vi "Swap CS with DDS.vi"(6 "Variant in":variant, 7 "Shift Pressed?":bool, 8 "error in (no error)":errorcluster, 10 "QD Combo Box Ref":refnum<vi>, 11 "QD Launch VI Ref":refnum<vi>) -> (0 "error out":errorcluster, 4 "Variant out":variant)   [LabVIEW 2017]
doc: "PLUGIN_DESCRIPTION: Replaces selected Case Structure with Diagram Disable Structure. Based on SAPHIR_DisableCode.vi from https://forums.ni.com/t5/SAPHIR-Toolkits-Documents/ViBox-Quick-Drop-datasheet/ta-p/3507939?profile.language=en\nPLUGIN_DEFAULT_SHORTCUT:"
uses:
  <userlib>/_LAVACR/Scripting Tools/Scripting Tools.lvlib
panel:
  in  "Undo Name":string="DisableCode"
  # "Created by https://github.com/Zieleslaw/, based on:"
  # "More informations on : https://decibel.ni.com/content/groups/saphir-toolkit"
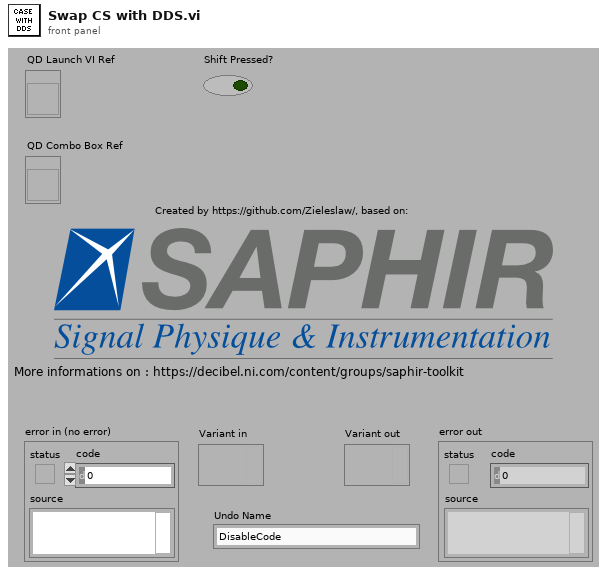
[diagram p1: front panel]
types:
  T1 = enum16{"Case Structure", "Stacked Sequence", "Event Structure", "Diagram Disable", "Conditional Disable", "While Loop", "For Loop", "Inplace Structure"}
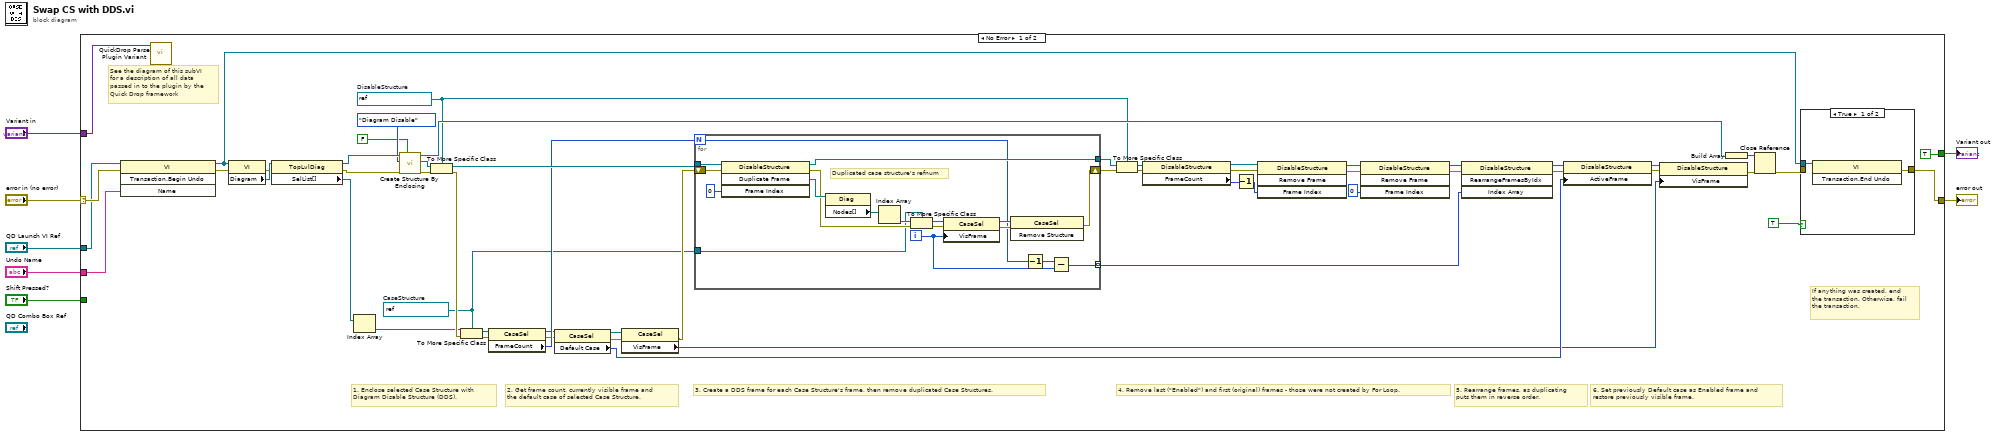
[diagram p0: block diagram]
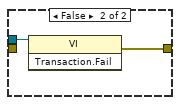
[diagram p2: hidden frame]
diagram:
  n1 = case shown="No Error" "error in (no error)" {
    selector: "error in (no error)" -> [w53 w85]
    tunnel: [w50 w85] -> w6
    tunnel: "QD Launch VI Ref" -> [w52 _]
    tunnel: "Variant in" -> [w54 _]
    tunnel: "Undo Name" -> [w51 _]
    tunnel: [TRUE _] -> w2
    tunnel: "Shift Pressed?" -> [_ _]
    frame No Error {
      w8 = refnum<vi> refnum  # CaseStructure
      w9 = refnum<vi> refnum  # DisableStructure
      # "6. Set previously Default case as Enabled frame and \nrestore previously visible frame."
      # "5. Rearrange frames, as duplicating \nputs them in reverse order."
      # "4. Remove last (\"Enabled\") and first (original) frames - those were not created by For Loop."
      # "3. Create a DDS frame for each Case Structure's frame, then remove duplicated Case Structures."
      # "2. Get frame count, currently visible frame and\nthe default case of selected Case Structure."
      # "1. Enclose selected Case Structure with\nDiagram Disable Structure (DDS)."
      # "If anything was created, end the transaction. Otherwise, fail the transaction."
      # "See the diagram of this subVI for a description of all data passed in to the plugin by the Quick Drop framework"
      n2 = invoke class="VI" method="Transaction.Begin Undo"(reference=w52, error in=w53, "Name"=w51) -> (reference out=w58:refnum<vi>, error out=w61:errorcluster)  [unwired: 1 in, 2 out]
      n3 = call <vilib>:"QuickDrop Parse Plugin Variant.vi"("QDKS Variant in"=w54) -> ()  [unwired: 12 in, 3 out]
      n4 = property class="VI"(reference=w58, error in=w61) -> (error out=w55:errorcluster, "Diagram"=w56:refnum<vi>)  [unwired: 1 out]
      n5 = property class="TopLvlDiag"(reference=w56, error in=w55) -> (reference out=w57:refnum<vi>, error out=w60:errorcluster, "SelList[]"=w48:refnum<vi>[])
      n6 = Index Array(array=w48) -> (element=w10:refnum<vi>)  [unwired: 1 in]
      n7 = call <userlib>:"Create Structure By Enclosing.vi"("Select everything except terminals ?"=FALSE, "error in (no error)"=w60, "Structure Type"=T1."Diagram Disable", "Diagram In"=w57) -> ("error out"=w44:errorcluster, "Structure Out"=w45:refnum<vi>, "Diagram Out"=w11:refnum<vi>)  [unwired: 5 in]
      n8 = To More Specific Class(target class=w9, reference=w45, error in=w44) -> (specific class reference=w42:refnum<vi>, error out=w32:errorcluster)
      n9 = To More Specific Class(target class=w8, reference=w10, error in=w32) -> (specific class reference=w40:refnum<vi>, error out=w33:errorcluster)
      n10 = property class="CaseSel"(reference=w40, error in=w33) -> (reference out=w38:refnum<vi>, error out=w37:errorcluster, "FrameCount"=w39:i32)
      n11 = property class="CaseSel"(reference=w38, error in=w37) -> (reference out=w35:refnum<vi>, error out=w34:errorcluster, "Default Case"=w36:i32)
      n12 = property class="CaseSel"(reference=w35, error in=w34) -> (error out=w12:errorcluster, "VisFrame"=w18:u32)  [unwired: 1 out]
      n13 = for {
        N: w39 -> [w67]
        tunnel: [w70] -> w30
        tunnel: w42 -> [w80]
        shift-right: [w71] -> w29
        shift-left: w12 -> [w79]
        tunnel: [w64] -> w17 mode=indexing
        tunnel: w8 -> [w63]
        i -> [w66]
        # "Duplicated case structure's refnum"
        n14 = invoke class="DisableStructure" method="Duplicate Frame"(reference=w80, error in=w79, "Frame Index"=u32 0) -> (reference out=w70:refnum<vi>, error out=w69:errorcluster, "Duplicate Frame"=w78:refnum<vi>)  [unwired: 1 in, 1 out]
        n15 = property class="Diag"(reference=w78) -> ("Nodes[]"=w77:refnum<vi>[])  [unwired: 1 in, 2 out]
        n16 = Index Array(array=w77) -> (element=w76:refnum<vi>)  [unwired: 1 in]
        n17 = To More Specific Class(target class=w63, reference=w76, error in=w69) -> (specific class reference=w75:refnum<vi>, error out=w74:errorcluster)
        n18 = property class="CaseSel"(reference=w75, error in=w74, "VisFrame"=w66) -> (reference out=w73:refnum<vi>, error out=w72:errorcluster)
        n19 = invoke class="CaseSel" method="Remove Structure"(reference=w73, error in=w72) -> (error out=w71:errorcluster)  [unwired: 1 in, 2 out]
        n20 = Decrement(x=w67) -> (x-1=w65:i32)
        n21 = Subtract(x=w65, y=w66) -> (x-y=w64:i32)
      }
      n22 = To More Specific Class(target class=w9, reference=w30, error in=w29) -> (specific class reference=w27:refnum<vi>, error out=w31:errorcluster)
      n23 = property class="DisableStructure"(reference=w27, error in=w31) -> (reference out=w26:refnum<vi>, error out=w28:errorcluster, "FrameCount"=w25:i32)
      n24 = Decrement(x=w25) -> (x-1=w22:i32)
      n25 = invoke class="DisableStructure" method="Remove Frame"(reference=w26, error in=w28, "Frame Index"=w22) -> (reference out=w24:refnum<vi>, error out=w23:errorcluster)  [unwired: 1 in, 2 out]
      n26 = invoke class="DisableStructure" method="Remove Frame"(reference=w24, error in=w23, "Frame Index"=u32 0) -> (reference out=w16:refnum<vi>, error out=w14:errorcluster)  [unwired: 1 in, 2 out]
      n27 = invoke class="DisableStructure" method="RearrangeFramesByIdx"(reference=w16, error in=w14, "Index Array"=w17) -> (reference out=w15:refnum<vi>, error out=w13:errorcluster)  [unwired: 1 in, 2 out]
      n28 = property class="DisableStructure"(reference=w15, error in=w13, "ActiveFrame"=w36) -> (reference out=w19:refnum<vi>, error out=w20:errorcluster)
      n29 = property class="DisableStructure"(reference=w19, error in=w20, "VisFrame"=w18) -> (error out=w43:errorcluster)  [unwired: 1 out]
      n30 = Build Array(w11) -> (w41:refnum<vi>[])
      n31 = Close Reference(reference=w41, error in (no error)=w43) -> (error out=w59:errorcluster)
      n32 = case shown="True" TRUE ("x") {
        tunnel: w58 -> [w81 w83]
        tunnel: [w82 w84] -> w50
        tunnel: w59 -> [_ _]
        frame True {
          n33 = invoke class="VI" method="Transaction.End Undo"(reference=w81) -> (error out=w82:errorcluster)  [unwired: 2 in, 2 out]
        }
        frame False {
          n34 = invoke class="VI" method="Transaction.Fail"(reference=w83) -> (error out=w84:errorcluster)  [unwired: 2 in, 2 out]
        }
      }
    }
    frame Error {
    }
  }
  "error out" <- w6
  "Variant out" <- w2
